vi "Untitled 2.vi"() -> ()   [LabVIEW 2018]
panel:
  in  "Play Button":bool=TRUE
  in  "stop":bool
  out "x = 0?":bool
  out "Numeric":i32
  out "Boolean":bool=TRUE
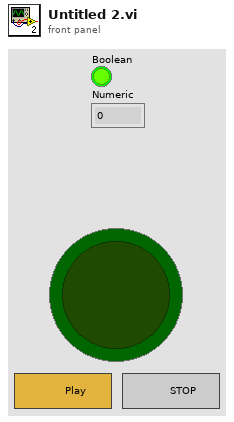
[diagram p1: front panel]
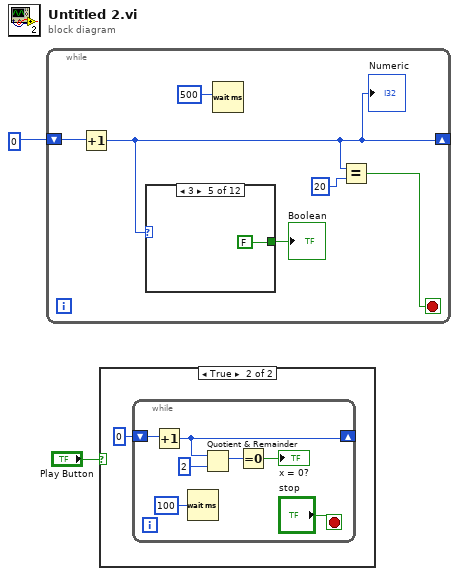
[diagram p0: block diagram]
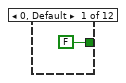
[diagram p3: hidden frame]
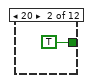
[diagram p4: hidden frame]
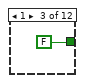
[diagram p5: hidden frame]
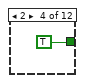
[diagram p6: hidden frame]
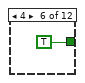
[diagram p7: hidden frame]
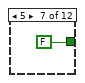
[diagram p8: hidden frame]
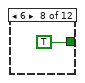
[diagram p9: hidden frame]
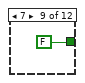
[diagram p10: hidden frame]
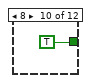
[diagram p11: hidden frame]
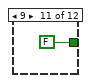
[diagram p12: hidden frame]
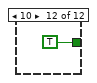
[diagram p13: hidden frame]
diagram:
  n1 = while {
    shift-right: [w4] -> _
    shift-left: 0 -> [w8]
    stop <- w3 stop-if-true
    n2 = Increment(x=w8) -> (x+1=w4:i32)
    "Numeric" <- w4
    n3 = case shown="3" w4 {
      tunnel: [FALSE TRUE FALSE TRUE FALSE TRUE FALSE TRUE FALSE TRUE FALSE TRUE] -> w7
      frame 0, Default {
      }
      frame 20 {
      }
      frame 1 {
      }
      frame 2 {
      }
      frame 3 {
      }
      frame 4 {
      }
      frame 5 {
      }
      frame 6 {
      }
      frame 7 {
      }
      frame 8 {
      }
      frame 9 {
      }
      frame 10 {
      }
    }
    "Boolean" <- w7
    n4 = Wait (ms)(milliseconds to wait=500) -> ()  [unwired: 1 out]
    n5 = Equal?(x=w4, y=20) -> (x = y?=w3:bool)
  }
  n6 = case shown="True" "Play Button" {
    frame False {
    }
    frame True {
      n7 = while {
        shift-right: [w25] -> _
        shift-left: 0 -> [w28]
        stop <- "stop" stop-if-true
        n8 = Increment(x=w28) -> (x+1=w25:i32)
        n9 = Wait (ms)(milliseconds to wait=u32 100) -> ()  [unwired: 1 out]
        n10 = Quotient & Remainder(x=w25, y=2) -> (x-y*floor(x/y)=w22:i32)  [unwired: 1 out]
        n11 = Equal To 0?(x=w22) -> (x = 0?=→"x = 0?":bool)
      }
    }
  }
